vi "Pack3.vi"(8 "ClusterIn":T2={"Header size"=56, "MagicWord"=305419896, "byte order"=enum."little-endian", "Проверка конца пакета"=TRUE, "Проверка CRC8"=TRUE, "LastPacketIn"=6858, "MinimalString"=10000} {"MagicWord" format="%.0x"}, 11 "StringIn":string) -> (0 "ClusterOut":T1, 2 "Array":T3(array[cluster]) {"Reserve3" format="%08x"; "OverloadSamplesChannelY" format="%04x"; "OverloadSamplesChannelX" format="%04x"; "SamplingInterval" format="%#_6e"; "LoseSamples" format="%08x"; "EncodersParam2" format="%016x"; "EncodersParam1" format="%016x"; "CRC 8" format="%02x"; "Reserve2" format="%02x"; "Reserve" format="%02x"; "Ncycle" format="%04x"; "FrameFormatVersion" format="%02x"; "MagicWord" format="%.0x"}, 3 "StringLast":string)   [LabVIEW 2017]
uses:
  Control_EU/ClusterPack (Type).ctl
panel:
  out "StringLast 2":string
  out "ErrorSizeCount":i32
  out "ErrorCRC8Count":i32
  out "ErrorCRC8":bool
  out "DataSize":u16
  out "Оставшиеся байты":u32
  out "offsetMagicWord":i32
  out "DataSizeSmall":bool
  out "ErrorEndPack":bool
  out "ErrorSeqPackCount":i32
  out "ErrorSequence":bool
  out "LastPacket":u32
  out "PackGoodParsing":i32
  out "Iteration":i32
  out "MagicWordStr":string
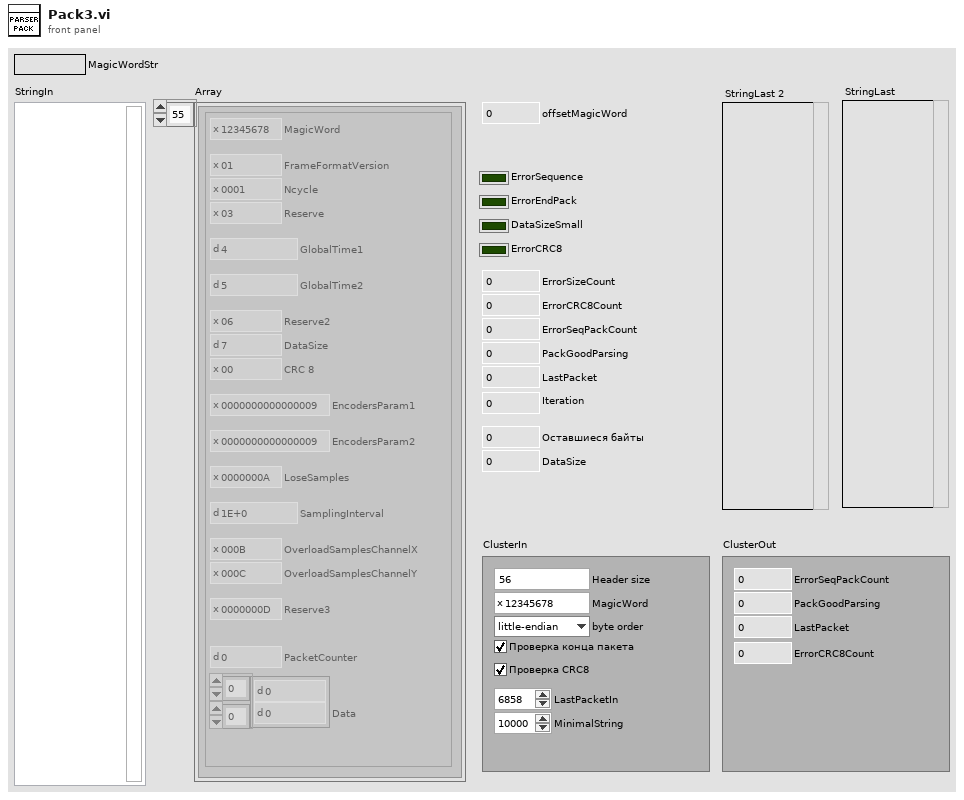
[diagram p1: front panel]
types:
  T1 = cluster{"PackGoodParsing":u32, "LastPacket":u32, "ErrorSeqPackCount":u32, "ErrorCRC8Count":u32}
  T2 = cluster{"Header size":u32, "MagicWord":u32, "byte order":enum16{"big-endian, network order", "native, host order", "little-endian"}, "Проверка конца пакета":bool, "Проверка CRC8":bool, "LastPacketIn":u32, "MinimalString":i32}
  T3 = cluster{"MagicWord":u32, "FrameFormatVersion":u8, "Ncycle":u16, "Reserve":u8, "GlobalTime1":u32, "GlobalTime2":u32, "Reserve2":u8, "DataSize":u16, "CRC 8":u8, "EncodersParam1":u64, "EncodersParam2":u64, "LoseSamples":u32, "SamplingInterval":sgl, "OverloadSamplesChannelX":u16, "OverloadSamplesChannelY":u16, "Reserve3":u32, "PacketCounter":u32, "Data":dbl[][]}[]
  T4 = typedef "ClusterPack (Type).ctl" = cluster{"MagicWord":u32, "FrameFormatVersion":u8, "Ncycle":u16, "Reserve":u8, "GlobalTime1":u32, "GlobalTime2":u32, "Reserve2":u8, "DataSize":u16, "CRC 8":u8, "EncodersParam1":u64, "EncodersParam2":u64, "LoseSamples":u32, "SamplingInterval":sgl, "OverloadSamplesChannelX":u16, "OverloadSamplesChannelY":u16, "Reserve3":u32, "PacketCounter":u32, "Data1":dbl[][]}
  T5 = enum16{"big-endian, network order", "native, host order", "little-endian"}
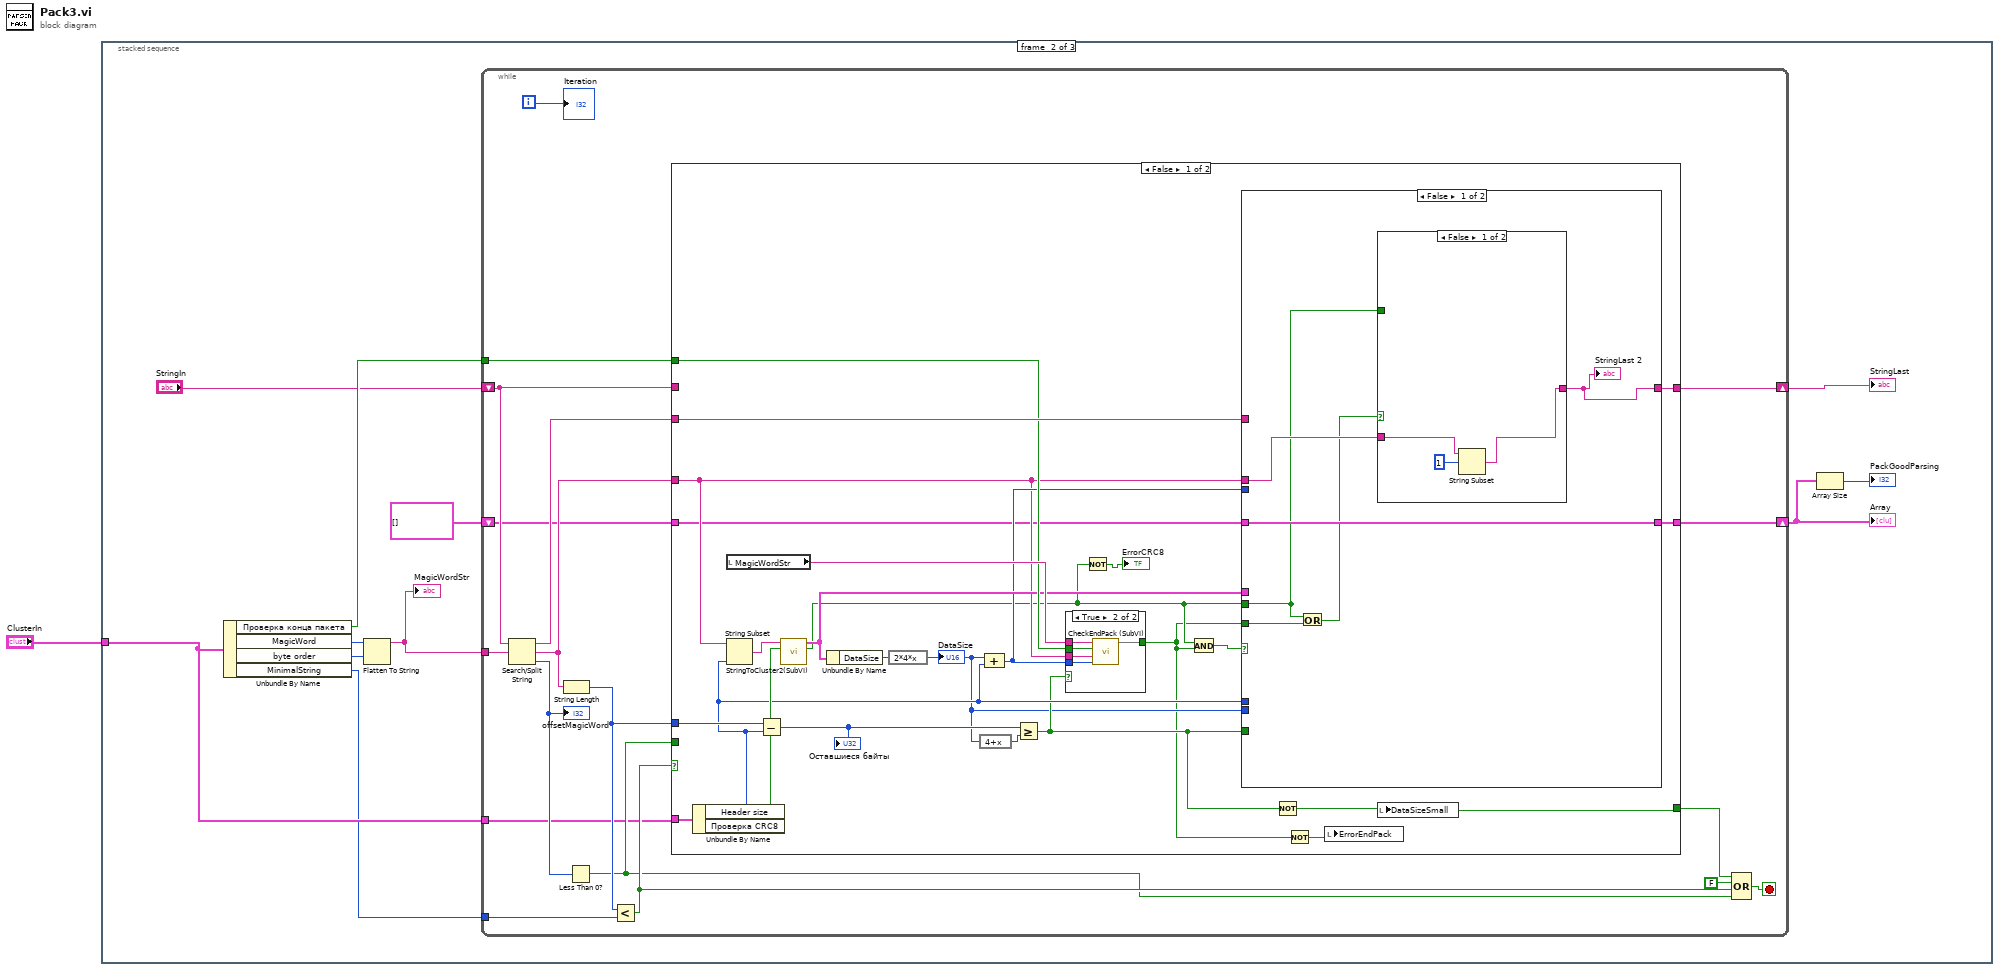
[diagram p0: block diagram]
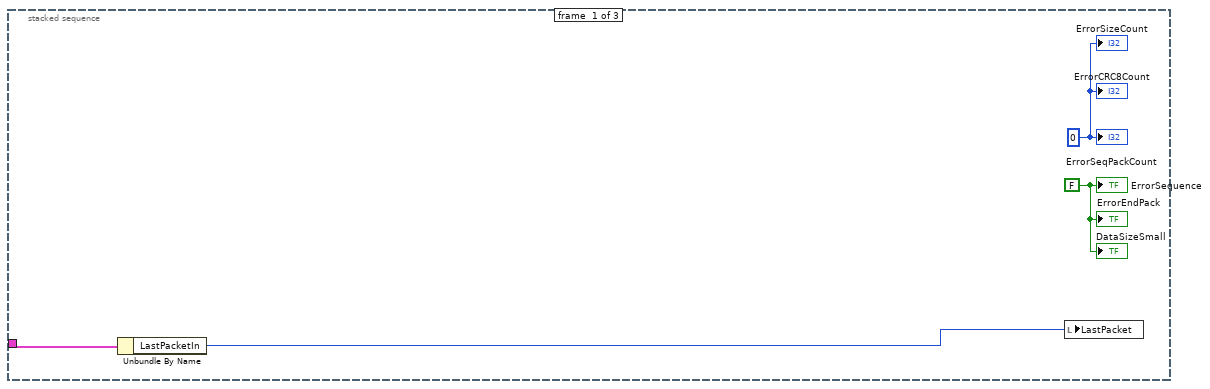
[diagram p2: hidden frame]
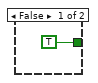
[diagram p3: hidden frame]
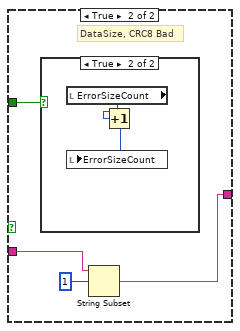
[diagram p4: hidden frame]
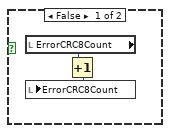
[diagram p5: hidden frame]
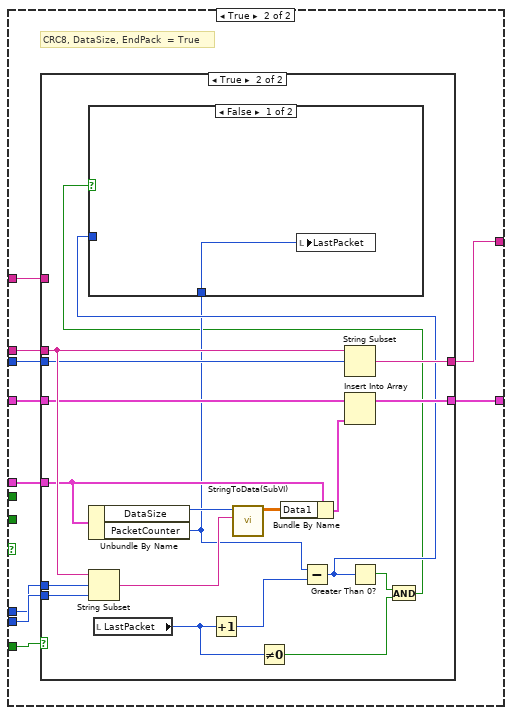
[diagram p6: hidden frame]
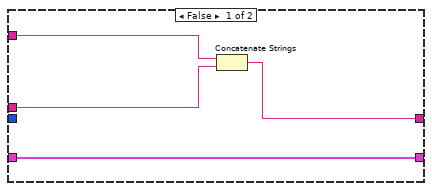
[diagram p7: hidden frame]
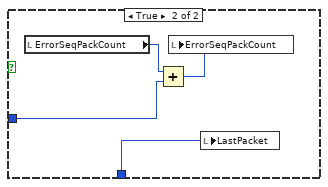
[diagram p8: hidden frame]
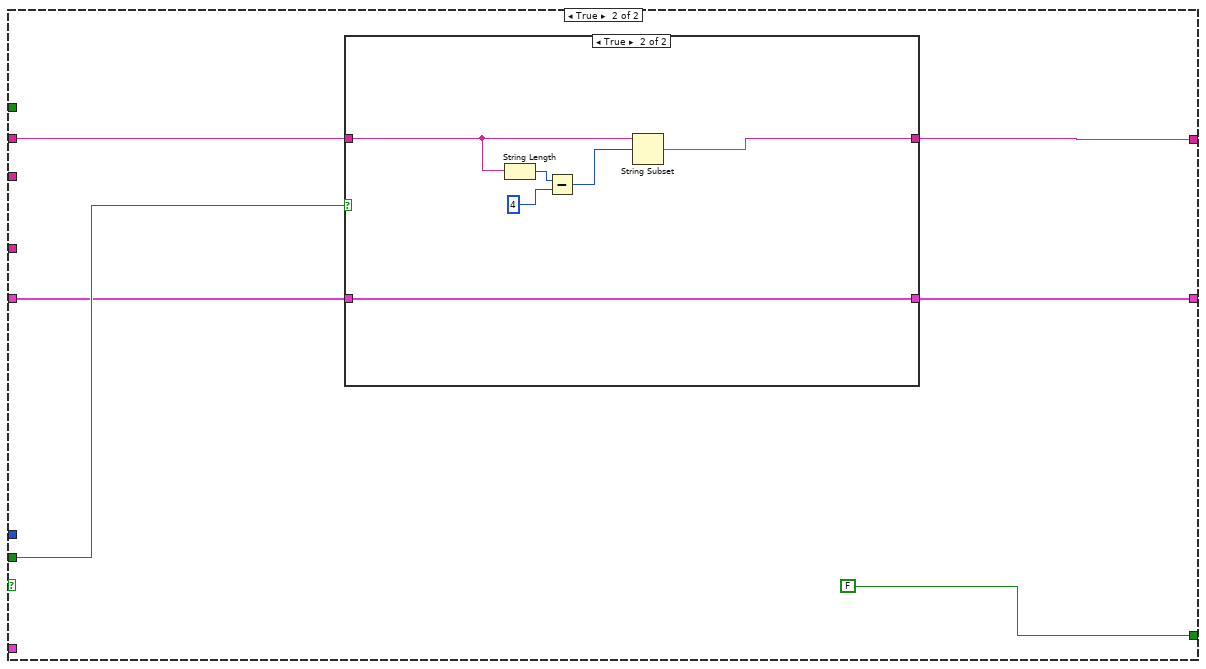
[diagram p9: hidden frame]
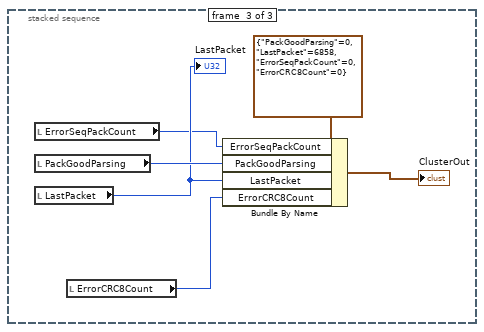
[diagram p11: hidden frame]
diagram:
  n1 = stacked-sequence {
    tunnel: "ClusterIn" -> [w5 w7 _]
    frame #0 {
      w2 = 0 ("ErrorSeqCount")
      w3 = FALSE ("PackLost")
      n2 = Unbundle By Name(w5) -> ("LastPacketIn"=w4:u32)
      n3 = local write "LastPacket"(w4) -> ()
      "ErrorSequence" <- w3
      "ErrorSeqPackCount" <- w2
      "ErrorEndPack" <- w3
      "ErrorCRC8Count" <- w2
      "DataSizeSmall" <- w3
      "ErrorSizeCount" <- w2
    }
    frame #1 {
      n4 = Unbundle By Name(w7) -> ("Проверка конца пакета"=w10:bool, "MagicWord"=w13:u32, "byte order"=w14:T5, "MinimalString"=w6:i32)
      n5 = Flatten To String(anything=w13, byte order (0:big-endian, network order)=w14) -> (data string=w16:string)  [unwired: 2 in, 2 out]
      "MagicWordStr" <- w16
      n6 = while {
        tunnel: w16 -> [w34]
        shift-right: [w17] -> w15
        shift-left: "StringIn" -> [w28]
        tunnel: w10 -> [w33]
        shift-right: [w24] -> w9
        shift-left: T4[] [] -> [w23]
        tunnel: w7 -> [w21]
        tunnel: w6 -> [w20]
        i -> [w25]
        stop <- w31 stop-if-true
        n7 = Search/Split String(string=w28, search string/char (-)=w34) -> (substring before match=w32:string, match + rest of string=w29:string, offset of match=w26:i32)  [unwired: 1 in]
        "offsetMagicWord" <- w26
        n8 = String Length(string=w29) -> (length=w27:i32)
        n9 = Less Than 0?(x=w26) -> (x < 0?=w22:bool)
        n10 = Less?(x=w27, y=w20) -> (x < y?=w30:bool)
        n11 = case shown="False" w30 {
          tunnel: w29 -> [w50 _]
          tunnel: [w59 w123] -> w17
          tunnel: w33 -> [w55 _]
          tunnel: [w36 FALSE] -> w18
          tunnel: w32 -> [w58 _]
          tunnel: w28 -> [_ w122]
          tunnel: w27 -> [w51 _]
          tunnel: w21 -> [w48 _]
          tunnel: [w45 w125] -> w24
          tunnel: w23 -> [w44 w124]
          tunnel: w22 -> [_ w126]
          frame False {
            n12 = Unbundle By Name(w48) -> ("Header size"=w46:u32, "Проверка CRC8"=w47:bool)
            n13 = local read "MagicWordStr"() -> (w56:string)
            n14 = String Subset(string=w50, length (rest)=w46) -> (substring=w49:string)  [unwired: 1 in]
            n15 = Subtract(x=w51, y=w46) -> (x-y=w42:u32)
            "Оставшиеся байты" <- w42
            n16 = call "StringToCluster2(SubVI).vi"("Проверка CRC8"=w47, "StringIn"=w49) -> ("CRC8Good"=w38:bool, "ECC_Cluster"=w54:T4)  [unwired: 8 in]
            n17 = Unbundle By Name(w54) -> ("DataSize"=w57:u16)
            n18 = expression code="2*4*x"(w57) -> (w40:u16)
            "DataSize" <- w40
            n19 = expression code="4+x"(w40) -> (w39:u16)
            n20 = Compound Arithmetic op=ADD(w40, w46) -> (w53:u32)
            n21 = Greater Or Equal?(x=w42, y=w39) -> (x >= y?=w43:bool)
            n22 = case shown="True" w43 {
              tunnel: w56 -> [_ w65]
              tunnel: w55 -> [_ w64]
              tunnel: w53 -> [_ w63]
              tunnel: w50 -> [_ w62]
              tunnel: [TRUE ("PackEndGood") w61] -> w35
              frame False {
              }
              frame True {
                n23 = call "CheckEndPack (SubVI).vi"("error in"=w63, "OfsetEndPack"=w62, 10:w64, "data"=w65) -> (3:w61)  [unwired: 4 in, 3 out]
              }
            }
            n24 = Not(x=w38) -> (.not. x?=→"ErrorCRC8":bool)
            n25 = Compound Arithmetic op=AND(w38, w35) -> (w52:bool)
            n26 = case shown="False" w52 {
              tunnel: [w67 w92] -> w59
              tunnel: w58 -> [_ w91]
              tunnel: w50 -> [w70 w90]
              tunnel: w54 -> [_ w89]
              tunnel: w40 -> [_ w88]
              tunnel: w46 -> [_ w87]
              tunnel: w53 -> [_ w86]
              tunnel: w43 -> [_ w85]
              tunnel: [w71 w84] -> w45
              tunnel: w44 -> [w71 w83]
              tunnel: w38 -> [w68 _]
              tunnel: w35 -> [w66 _]
              frame False {
                n27 = Or(x=w68, y=w66) -> (x .or. y?=w69:bool)
                n28 = case shown="False" w69 {
                  tunnel: [w72 w75] -> w67
                  tunnel: w70 -> [w73 w76]
                  tunnel: w68 -> [_ w78]
                  frame False {
                    n29 = String Subset(string=w73, offset (0)=1) -> (substring=w72:string)  [unwired: 1 in]
                  }
                  frame True {
                    # "DataSize, CRC8 Bad"
                    n30 = case shown="True" w78 {
                      frame False {
                        n31 = local read "ErrorCRC8Count"() -> (w80:i32)
                        n32 = Increment(x=w80) -> (x+1=w79:i32)
                        n33 = local write "ErrorCRC8Count"(w79) -> ()
                      }
                      frame True {
                        n34 = local read "ErrorSizeCount"() -> (w82:i32)
                        n35 = Increment(x=w82) -> (x+1=w81:i32)
                        n36 = local write "ErrorSizeCount"(w81) -> ()
                      }
                    }
                    n37 = String Subset(string=w76, offset (0)=1) -> (substring=w75:string)  [unwired: 1 in]
                  }
                }
                "StringLast 2" <- w67
              }
              frame True {
                # "CRC8, DataSize, EndPack  = True"
                n38 = case shown="True" w85 {
                  tunnel: w89 -> [_ w109]
                  tunnel: [w94 w111] -> w92
                  tunnel: w87 -> [_ w113]
                  tunnel: w90 -> [w96 w110]
                  tunnel: w88 -> [_ w112]
                  tunnel: w91 -> [w95 _]
                  tunnel: w86 -> [_ w107]
                  tunnel: [w93 w105] -> w84
                  tunnel: w83 -> [w93 w104]
                  frame False {
                    n39 = Concatenate Strings(w95, w96) -> (w94:string)
                  }
                  frame True {
                    n40 = Unbundle By Name(w109) -> ("DataSize"=w108:u16, "PacketCounter"=w101:u32)
                    n41 = String Subset(string=w110, offset (0)=w113, length (rest)=w112) -> (substring=w114:string)
                    n42 = local read "LastPacket"() -> (w98:u32)
                    n43 = Increment(x=w98) -> (x+1=w103:u32)
                    n44 = call "StringToData(SubVI).vi"("StringIn"=w114, "DataSize"=w108) -> ("DataOut"=w115:dbl[][])  [unwired: 9 in]
                    n45 = Not Equal To 0?(x=w98) -> (x != 0?=w97:bool)
                    n46 = Bundle By Name(cluster=w109, "Data1"=w115) -> (w106:T4)
                    n47 = Subtract(x=w101, y=w103) -> (x-y=w102:u32)
                    n48 = String Subset(string=w110, offset (0)=w107) -> (substring=w111:string)  [unwired: 1 in]
                    n49 = Insert Into Array(array=w104, new element=w106) -> (w105:T4[])  [unwired: 1 in]
                    n50 = Greater Than 0?(x=w102) -> (x > 0?=w100:bool)
                    n51 = And(x=w100, y=w97) -> (x .and. y?=w99:bool)
                    n52 = case shown="False" w99 {
                      tunnel: w102 -> [_ w118]
                      tunnel: w101 -> [w116 w117]
                      frame False {
                        n53 = local write "LastPacket"(w116) -> ()
                      }
                      frame True {
                        n54 = local read "ErrorSeqPackCount"() -> (w120:i32)
                        n55 = Add(x=w120, y=w118) -> (x+y=w119:u32)
                        n56 = local write "ErrorSeqPackCount"(w119) -> ()
                        n57 = local write "LastPacket"(w117) -> ()
                      }
                    }
                  }
                }
              }
            }
            n58 = Not(x=w43) -> (.not. x?=w36:bool)
            n59 = Not(x=w35) -> (.not. x?=w41:bool)
            n60 = local write "ErrorEndPack"(w41) -> ()
            n61 = local write "DataSizeSmall"(w36) -> ()
          }
          frame True {
            n62 = case shown="True" w126 {
              tunnel: [w127 w134] -> w125
              tunnel: w124 -> [w127 w134]
              tunnel: [w128 w129] -> w123
              tunnel: w122 -> [w128 w133]
              frame False {
              }
              frame True {
                n63 = String Length(string=w133) -> (length=w132:i32)
                n64 = Subtract(x=w132, y=4) -> (x-y=w130:i32)
                n65 = String Subset(string=w133, offset (0)=w130) -> (substring=w129:string)  [unwired: 1 in]
              }
            }
          }
        }
        n66 = Compound Arithmetic op=OR(w18, FALSE ("value"), w30, w22) -> (w31:bool)
        "Iteration" <- w25
      }
      "StringLast" <- w15
      "Array" <- w9
      n67 = Array Size(array=w9) -> (size(s)=→"PackGoodParsing":i32)
    }
    frame #2 {
      n68 = local read "ErrorSeqPackCount"() -> (w136:i32)
      n69 = local read "PackGoodParsing"() -> (w138:i32)
      n70 = local read "LastPacket"() -> (w137:u32)
      "LastPacket" <- w137
      n71 = local read "ErrorCRC8Count"() -> (w135:i32)
      n72 = Bundle By Name(cluster=T1 {"PackGoodParsing"=0, "LastPacket"=6858, "ErrorSeqPackCount"=0, "ErrorCRC8Count"=0} ("ClusterOut"), "ErrorSeqPackCount"=w136, "PackGoodParsing"=w138, "LastPacket"=w137, "ErrorCRC8Count"=w135) -> (→"ClusterOut":T1)
    }
  }
